vi "IPI_ReadINI.vi"(7 "名称或相对路径":string="UserDefine.ini", 10 "Keys":string[](array[string])=["LoadProgram"], 11 "section":string="BaseParam_Set") -> (3 "Outputs":string[](array[string]))   [LabVIEW 2015]
uses:
  Global System.vi
  <vilib>/Utility/config.llb/NI_LVConfig.lvlib
panel:
  out "error out":errorcluster caption="错误输出"
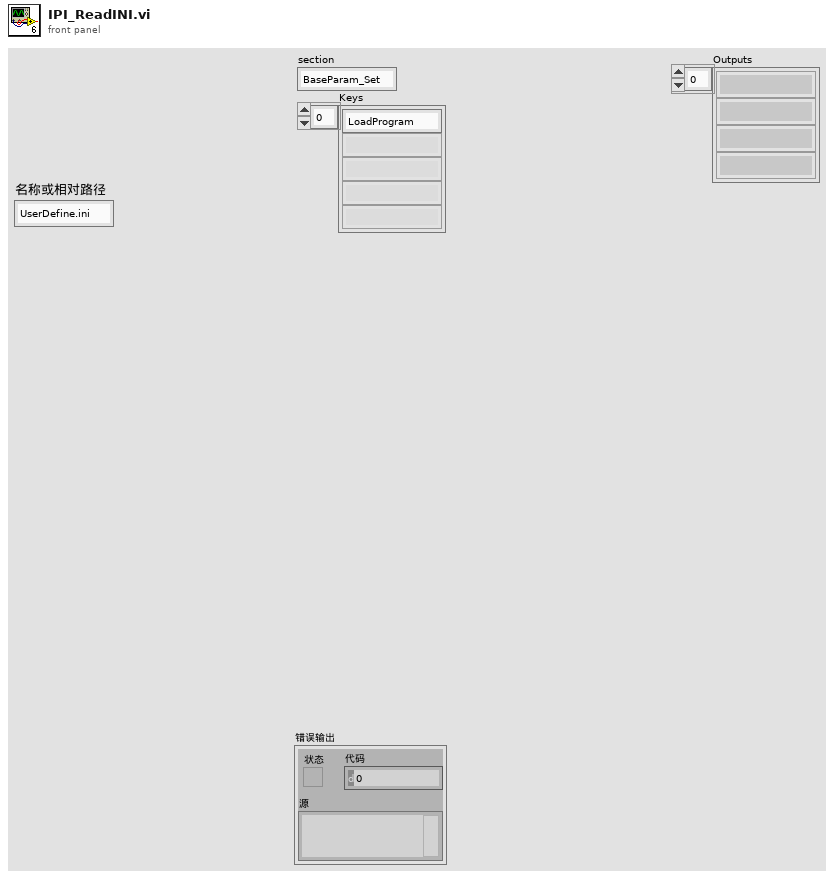
[diagram p1: front panel]
types:
  T1 = typedef "NI_LVConfig.lvlib/Config Data RefNum.ctl" = refnum<k1>
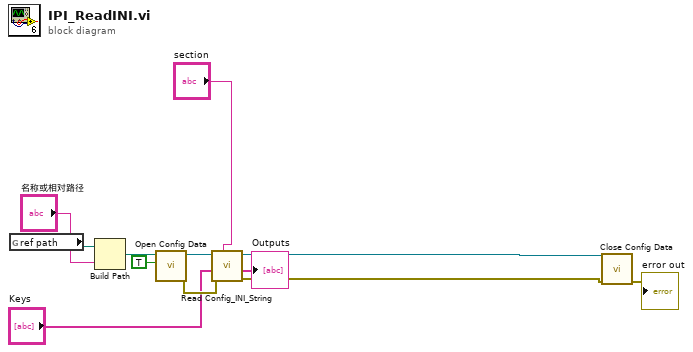
[diagram p0: block diagram]
diagram:
  n1 = global read "Global System.vi" "ref path"() -> (w6:path)
  n2 = Build Path(base path=w6, name or relative path="名称或相对路径") -> (appended path=w9:path)
  n3 = call <vilib>:"Open Config Data.vi"("create file if necessary (T)"=TRUE, "configuration file path"=w9) -> ("error out"=w11:errorcluster, "refnum"=w10:T1)  [unwired: 7 in, 1 out]
  n4 = call "Read Config_INI_String.vi"("section"="section", "error in (no error)"=w11, "Keys"="Keys", "refnum"=w10) -> ("error out"=w2:errorcluster, "Outputs"=→"Outputs":string[], "refnum out"=w3:T1)  [unwired: 5 in]
  n5 = call <vilib>:"Close Config Data.vi"("error in (no error)"=w2, "refnum"=w3) -> ("error out"=→"error out":errorcluster)  [unwired: 8 in, 1 out]
